vi "读取内置参数.vi"(8 "error in (no error)":errorcluster, 11 "MB session in":refnum<class "MB_Master.lvclass">) -> (0 "error out":errorcluster, 1 "float":T1 {"偏心轮校准参数" format="%#.6g"}, 2 "外设配置":T3 {"阀数量" items=["9通"=9, "12通"=12]; "泵类型" items=["TECAN", "润泽"]}, 3 "MB session out":refnum<class "MB_Master.lvclass">, 5 "量程参数读取":T2 {"阈值（高->低）" format="%#.6g"; "阈值（低->高）" format="%#.6g"; "下限" format="%#.6g"; "上限" format="%#.6g"})   [LabVIEW 2016, in "斯坦道CODMn新电路板.lvlib"]
uses:
  <vilib>/Plasmionique/MB Master/MB_Master/MB_Master.lvclass
  <vilib>/Plasmionique/MB Master/MB_Master_Serial/MB_Master_Serial.lvclass
  D:/Program Files (x86)/National Instruments/LabVIEW 2016/vi.lib/Plasmionique/MB Master/MB_Master/MB_Master.lvclass
  <vilib>/Plasmionique/MB Master/MB Master.lvlib
panel:
  in  "VISA Resource":refnum<visa-resource-name>
  in  "引用选择":enum16{"MB引用", "自建引用"}(ring)
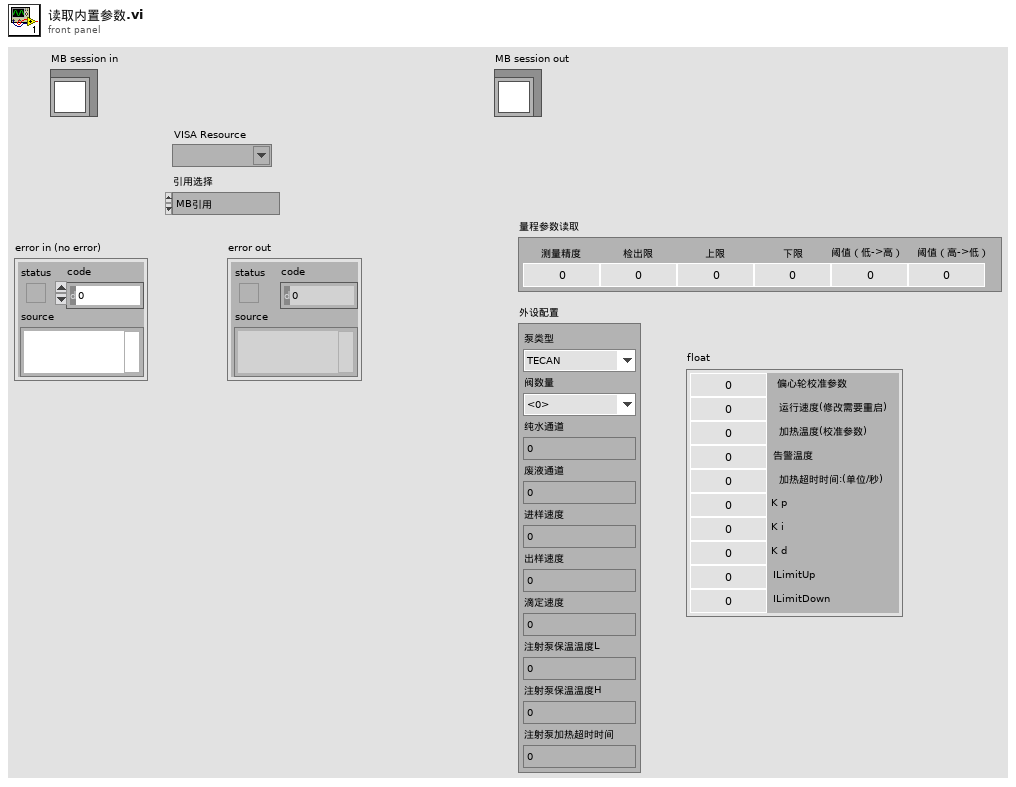
[diagram p1: front panel]
types:
  T1 = cluster{"偏心轮校准参数":dbl, "运行速度(修改需要重启)":u16, "加热温度(校准参数) ":dbl, "告警温度":dbl, "加热超时时间:(单位/秒)":dbl, "K p":dbl, "K i":dbl, "K d":dbl, "ILimitUp":dbl, "ILimitDown":dbl}
  T2 = cluster{"测量精度":dbl, "检出限":dbl, "上限":dbl, "下限":dbl, "阈值（低->高）":dbl, "阈值（高->低）":dbl}
  T3 = cluster{"泵类型":u8, "阀数量":u8, "纯水通道":u8, "废液通道":u8, "进样速度":u16, "出样速度":u16, "滴定速度":u16, "注射泵保温温度L":u8, "注射泵保温温度H":u8, "注射泵加热超时时间":u16}
  T4 = cluster{"baud rate (bps)":u32, "stop bits":u16, "parity":u16, "flow control":u16, "timeout":u32, "retries":i32}
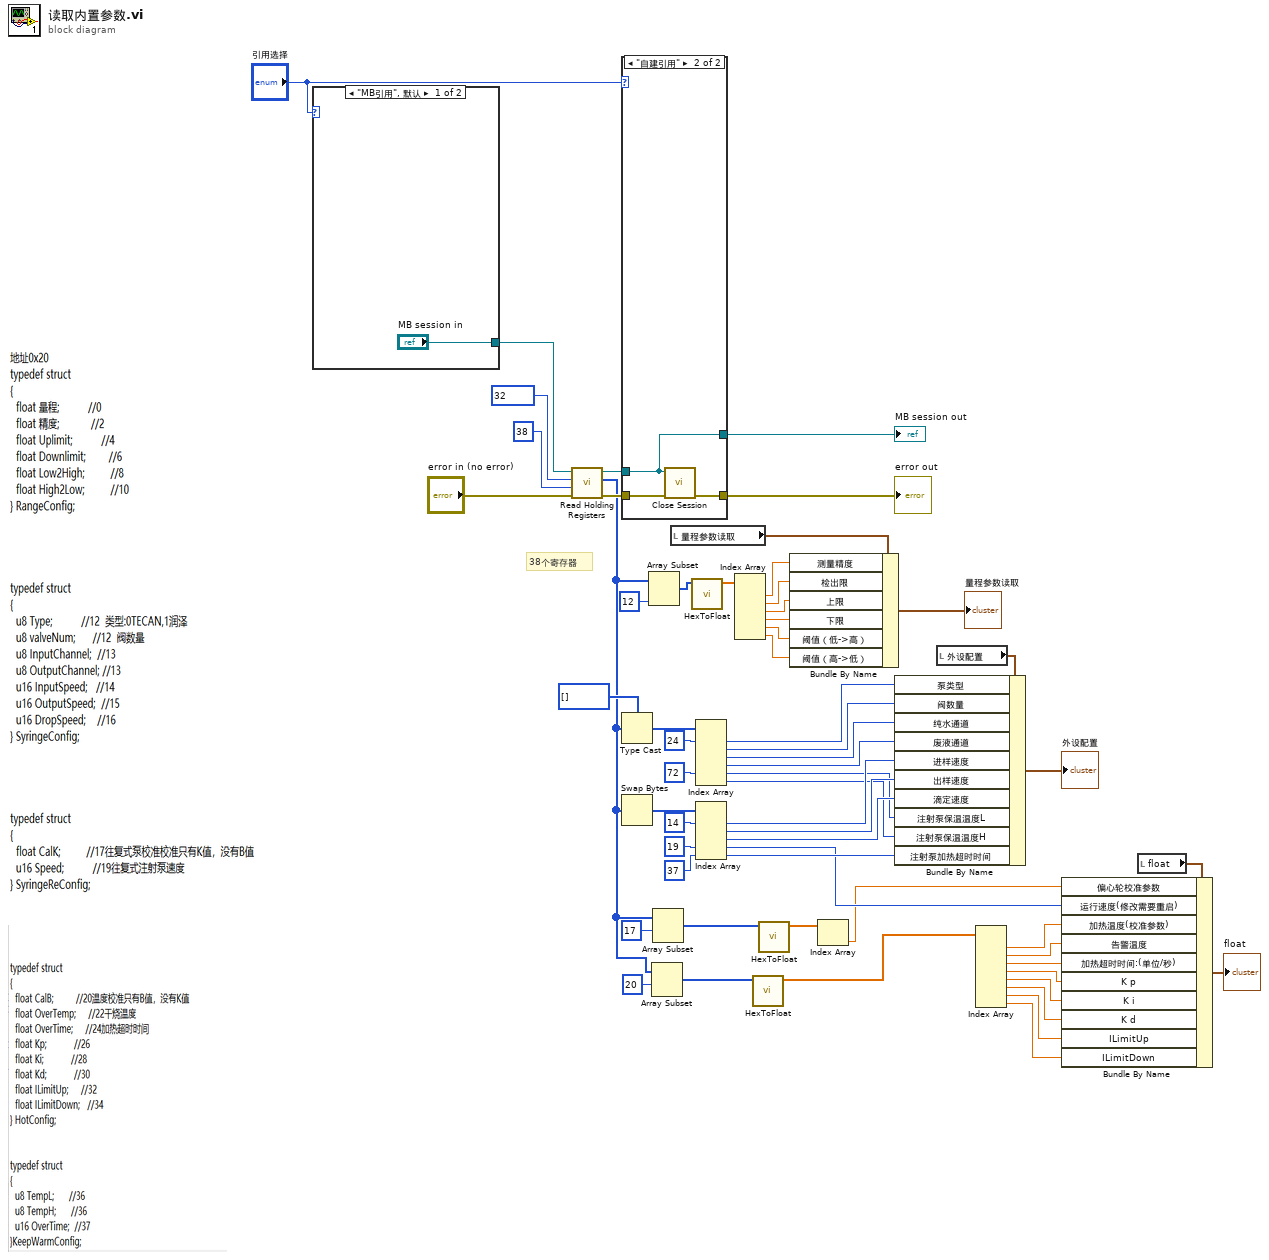
[diagram p0: block diagram]
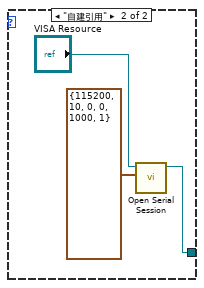
[diagram p3: hidden frame]
diagram:
  # "38个寄存器"
  n1 = case shown="\"MB引用\", 默认" "引用选择" {
    tunnel: ["MB session in" w63] -> w51
    frame "MB引用", Default {
    }
    frame "自建引用" {
      n2 = call <vilib>:"Open Serial Session.vi"("Serial Config"=T4 {"baud rate (bps)"=115200, "stop bits"=10, "parity"=0, "flow control"=0, "timeout"=1000, "retries"=1}, "VISA Resource"="VISA Resource") -> ("MB_Serial session"=w63:refnum<class "MB_Master_Serial.lvclass">)  [unwired: 8 in, 1 out]
    }
  }
  n3 = call <vilib>:"Read Holding Registers.vi"("error in (no error)"="error in (no error)", "quantity"=u16 38, "starting address"=u16 32, "MB session in"=w51) -> ("error out"=w48:errorcluster, "Registers"=w5:u16[], "MB session out"=w50:refnum<class "MB_Master.lvclass">)  [unwired: 5 in]
  n4 = case shown="\"自建引用\"" "引用选择" {
    tunnel: w50 -> [w64 w66]
    tunnel: w48 -> [w65 w68]
    tunnel: [w65 w67] -> w47
    tunnel: [w64 w66] -> w46
    frame "MB引用", Default {
    }
    frame "自建引用" {
      n5 = call-dynamic "Close Session.vi"("error in (no error)"=w68, "MB session in"=w66) -> ("error out"=w67:errorcluster)  [unwired: 9 in]
    }
  }
  "MB session out" <- w46
  "error out" <- w47
  n6 = Type Cast(type=u8[] [], x=w5) -> (*(type *) &x=w52:u8[])
  n7 = Swap Bytes(anything=w5) -> (byte swapped=w25:u16[])
  n8 = Array Subset(array=w5, length=12 ("长度")) -> (w7:u16[])  [unwired: 1 in]
  n9 = Array Subset(array=w5, index=20 ("索引")) -> (w4:u16[])  [unwired: 1 in]
  n10 = Array Subset(array=w5, index=17 ("索引")) -> (w18:u16[])  [unwired: 1 in]
  n11 = local read "量程参数读取"() -> (w44:T2)
  n12 = call "HexToFloat.vi"("数组"=w7) -> ("FLOAT"=w45:sgl[])  [unwired: 10 in]
  n13 = Index Array(array=w52, index #1=24 ("索引"), index #5=72 ("索引")) -> (element #1=w53:u8, element #2=w36:u8, element #3=w35:u8, element #4=w34:u8, element #5=w29:u8, element #6=w28:u8)  [unwired: 4 in]
  n14 = Index Array(array=w25, index #1=14 ("索引"), index #4=19 ("索引"), index #5=37 ("索引")) -> (element #1=w33:u16, element #2=w32:u16, element #3=w31:u16, element #4=w17:u16, element #5=w22:u16)  [unwired: 2 in]
  n15 = Index Array(array=w45) -> (element #1=w42:sgl, element #2=w41:sgl, element #3=w40:sgl, element #4=w39:sgl, element #5=w38:sgl, element #6=w37:sgl)  [unwired: 6 in]
  n16 = call "HexToFloat.vi"("数组"=w4) -> ("FLOAT"=w3:sgl[])  [unwired: 10 in]
  n17 = call "HexToFloat.vi"("数组"=w18) -> ("FLOAT"=w2:sgl[])  [unwired: 10 in]
  n18 = Bundle By Name(cluster=w44, "测量精度"=w42, "检出限"=w41, "上限"=w40, "下限"=w39, "阈值（低->高）"=w38, "阈值（高->低）"=w37) -> (→"量程参数读取":T2)
  n19 = Index Array(array=w2) -> (element=w1:sgl)  [unwired: 1 in]
  n20 = local read "外设配置"() -> (w55:T3)
  n21 = Bundle By Name(cluster=w55, "泵类型"=w53, "阀数量"=w36, "纯水通道"=w35, "废液通道"=w34, "进样速度"=w33, "出样速度"=w32, "滴定速度"=w31, "注射泵保温温度L"=w29, "注射泵保温温度H"=w28, "注射泵加热超时时间"=w22) -> (→"外设配置":T3)
  n22 = Index Array(array=w3) -> (element #1=w16:sgl, element #2=w15:sgl, element #3=w14:sgl, element #4=w13:sgl, element #5=w12:sgl, element #6=w11:sgl, element #7=w10:sgl, element #8=w9:sgl)  [unwired: 8 in]
  n23 = local read "float"() -> (w21:T1)
  n24 = Bundle By Name(cluster=w21, "偏心轮校准参数"=w1, "运行速度(修改需要重启)"=w17, "加热温度(校准参数)"=w16, "告警温度"=w15, "加热超时时间:(单位/秒)"=w14, "K p"=w13, "K i"=w12, "K d"=w11, "ILimitUp"=w10, "ILimitDown"=w9) -> (→"float":T1)
